vi "Create Wheel Angular Velocity Row.vi"(8 "error in (no error)":errorcluster, 10 "steering angle (rad)":dbl, 11 "wheel in":refnum<class "NI_Robotics_Wheel.lvclass">) -> (0 "error out":errorcluster, 2 "wheel angular velocity row":dbl[](array[numeric]), 3 "wheel out":refnum<class "NI_Robotics_Wheel.lvclass">)   [LabVIEW 2017, in "NI_Robotics_Wheel.lvclass"]
uses:
  <vilib>/robotics/Steering/Wheel/NI_Robotics_Wheel.lvclass
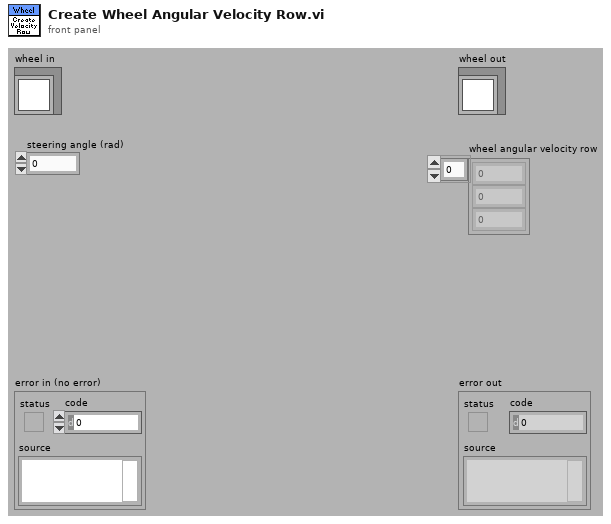
[diagram p1: front panel]
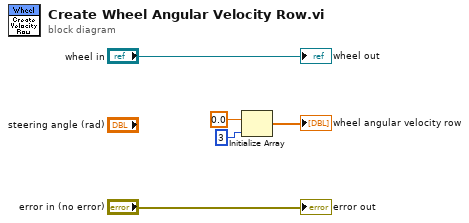
[diagram p0: block diagram]
diagram:
  n1 = Initialize Array(0.0 ("element"), 3 ("dimension size")) -> (→"wheel angular velocity row":dbl[])
  "error out" <- "error in (no error)"
  "wheel out" <- "wheel in"
